vi "getInheritanceChain.vi"(8 "error in (no error)":errorcluster, 11 "Structure in":refnum<class "Structure.lvclass">) -> (0 "error out":errorcluster, 2 "Inheritance Chain":string[](array[string]), 3 "Structure out":refnum<class "Structure.lvclass">)   [LabVIEW 2009, in "Structure.lvclass"]
doc: "Returns the inheritance chain."
uses:
  Structure.lvclass
  DataObj/DataObj.lvclass
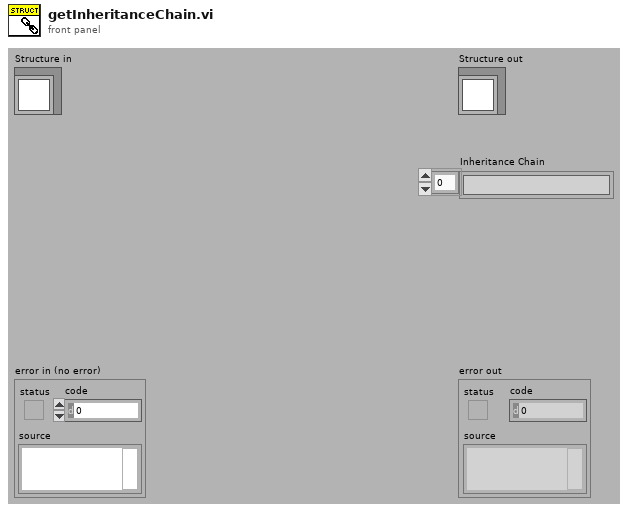
[diagram p1: front panel]
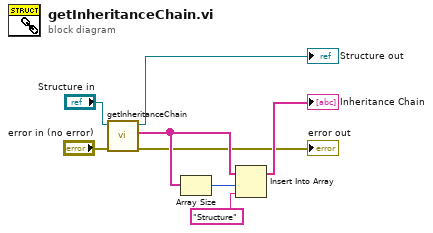
[diagram p0: block diagram]
diagram:
  n1 = call-parent "getInheritanceChain.vi"("error in (no error)"="error in (no error)", "DataObj in"="Structure in") -> ("error out"=→"error out":errorcluster, "Inheritance Chain"=w4:string[], "DataObj out"=→"Structure out":refnum<class "Structure.lvclass">)  [unwired: 7 in]
  n2 = Array Size(array=w4) -> (size(s)=w6:i32)
  n3 = Insert Into Array(array=w4, index=w6, new element="Structure") -> (→"Inheritance Chain":string[])
